vi "Start Sync.vi"(8 "error in":errorcluster, 10 "measurement plugin service in":refnum<class "Measurement Plugin Service.lvclass">, 11 "measurement service v1 in":refnum<class "Measurement Service V1.lvclass">) -> (0 "error out":errorcluster, 3 "measurement service v1 out":refnum<class "Measurement Service V1.lvclass">)   [LabVIEW 2020, in "Measurement Plugin Measurement Server.lvlib" / "Measurement Service V1.lvclass"]
uses:
  Measurement Service V1.lvclass
  C:/dev/measurementlink-labview/Source/Runtime/Measurement Plugin Measurement Server/IMeasurement Service/IMeasurement Service.lvclass
  Measurement Plugin Service/Measurement Plugin Service.lvclass
  Measurement Service V1.lvclass/Measurement Service V1.ctl
  Measurement Plugin Measurement Server Internal/RPC Service/MeasurementService/MeasurementServiceBaseV1.lvclass
  IMeasurement Service/IMeasurement Service.lvclass
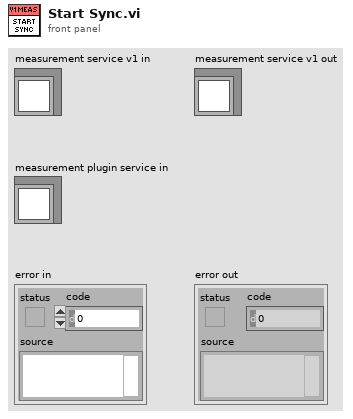
[diagram p1: front panel]
types:
  T1 = typedef "grpc-lvsupport-release.lvlib/grpcId.ctl" = u64
  T2 = typedef "Measurement Plugin Measurement Server.lvlib/Get Metadata Response.ctl" = cluster{"measurement details":T3, "measurement signature":T4, "user interface details":T9[]}
  T3 = typedef "Measurement Plugin Measurement Server.lvlib/Measurement Details.ctl" = cluster{"display name":string, "version":string}
  T4 = typedef "Measurement Plugin Measurement Server.lvlib/Measurement Signature.ctl" = cluster{"configuration parameters message type":string, "configuration parameters":T5[], "configuration defaults":T7, "outputs message type":string, "outputs":T8[]}
  T5 = typedef "Measurement Plugin Measurement Server.lvlib/Configuration Parameter.ctl" = cluster{"field number":i32, "type":i32, "name":string, "repeated":bool, "annotations":T6[], "message type":string}
  T6 = typedef "Measurement Plugin Measurement Server.lvlib/Parameter Annotations Entry.ctl" = cluster{"key":string, "value":string}
  T7 = typedef "grpc-lvsupport-release.lvlib/Any.ctl" = cluster{"Type Url":string, "Bytes":u8[]}
  T8 = typedef "Measurement Plugin Measurement Server.lvlib/Output Parameter.ctl" = cluster{"field number":i32, "type":i32, "name":string, "repeated":bool, "annotations":T6[], "message type":string}
  T9 = typedef "Measurement Plugin Measurement Server.lvlib/User Interface Details.ctl" = cluster{"file url":string}
  T10 = typedef "Measurement Plugin Measurement Server Internal.lvlib/ni_measurementlink_measurement_v1_GetMetadataResponse.ctl" = cluster{"measurement_details":T11, "measurement_signature":T12, "user_interface_details":T18[]}
  T11 = typedef "Measurement Plugin Measurement Server Internal.lvlib/ni_measurementlink_measurement_v1_MeasurementDetails.ctl" = cluster{"display_name":string, "version":string}
  T12 = typedef "Measurement Plugin Measurement Server Internal.lvlib/ni_measurementlink_measurement_v1_MeasurementSignature.ctl" = cluster{"configuration_parameters_message_type":string, "configuration_parameters":T13[], "configuration_defaults":T16, "outputs_message_type":string, "outputs":T17[]}
  T13 = typedef "Measurement Plugin Measurement Server Internal.lvlib/ni_measurementlink_measurement_v1_ConfigurationParameter.ctl" = cluster{"field_number":i32, "type":T14, "name":string, "repeated":bool, "annotations":T15[]}
  T14 = typedef "Measurement Plugin Measurement Server Internal.lvlib/google_protobuf_Field_Kind.ctl" = enum32{"TYPE_UNKNOWN", "TYPE_DOUBLE", "TYPE_FLOAT", "TYPE_INT64", "TYPE_UINT64", "TYPE_INT32", "TYPE_FIXED64", "TYPE_FIXED32", "TYPE_BOOL", "TYPE_STRING", "TYPE_GROUP", "TYPE_MESSAGE", "TYPE_BYTES", "TYPE_UINT32", "TYPE_ENUM", "TYPE_SFIXED32", "TYPE_SFIXED64", "TYPE_SINT32", "TYPE_SINT64"}
  T15 = typedef "Measurement Plugin Measurement Server Internal.lvlib/ni_measurementlink_measurement_v1_ConfigurationParameter_AnnotationsEntry.ctl" = cluster{"key":string, "value":string}
  T16 = typedef "Measurement Plugin Measurement Server Internal.lvlib/google_protobuf_Any.ctl" = cluster{"type_url":string, "value":u8[]}
  T17 = typedef "Measurement Plugin Measurement Server Internal.lvlib/ni_measurementlink_measurement_v1_Output.ctl" = cluster{"field_number":i32, "type":T14, "name":string, "repeated":bool}
  T18 = typedef "Measurement Plugin Measurement Server Internal.lvlib/ni_measurementlink_measurement_v1_UserInterfaceDetails.ctl" = cluster{"file_url":string}
  T19 = typedef "Measurement Plugin Measurement Server Internal.lvlib/ni_measurementlink_measurement_v1_MeasureRequest.ctl" = cluster{"configuration_parameters":T16, "pin_map_context":T20}
  T20 = typedef "Measurement Plugin Measurement Server Internal.lvlib/ni_measurementlink_PinMapContext.ctl" = cluster{"pin_map_id":string, "sites":i32[]}
  T21 = typedef "Measurement Plugin Measurement Server.lvlib/Measure Response.ctl" = cluster{"outputs":T16}
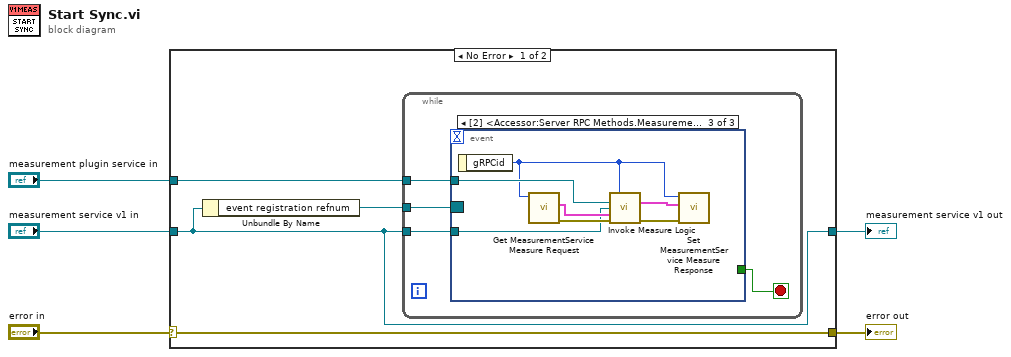
[diagram p0: block diagram]
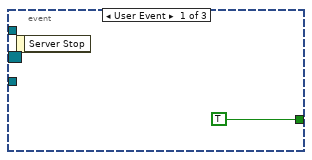
[diagram p2: hidden frame]
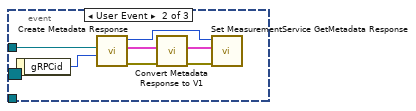
[diagram p3: hidden frame]
diagram:
  n1 = case shown="No Error" "error in" {
    selector: "error in" -> [w6 w30]
    tunnel: [w6 w30] -> w3
    tunnel: "measurement plugin service in" -> [w9 _]
    tunnel: "measurement service v1 in" -> [w8 w29]
    tunnel: [w8 w29] -> w1
    frame No Error {
      n2 = Unbundle By Name(w8) -> ("event registration refnum"=w7:refnum<event-registration>)
      n3 = while {
        tunnel: w7 -> [w13]
        tunnel: w9 -> [w12]
        tunnel: w8 -> [w10]
        stop <- w11 stop-if-true
        n4 = event "RPC Methods Event Structure" shown="[2] <Accessor:Server RPC Methods.MeasurementService Measure gRPC UE>: User Event" {
          selector: w13 -> [_ _ _]
          dyn-events: _ -> [_ _ _]
          timeout: _ -> [_ _ _]
          tunnel: [TRUE _ _] -> w11
          tunnel: w12 -> [_ w19 w27]
          tunnel: w10 -> [_ _ w22]
          event User Event {
            n5 = event-data() -> ()  [unwired: 1 in, 1 out]
          }
          event User Event {
            n6 = event-data() -> ("gRPCid"=w20:T1)  [unwired: 1 in]
            n7 = call "Create Metadata Response.vi"("gRPC ID"=w20, "measurement plugin service in"=w19) -> ("error out"=w18:errorcluster, "get metadata response"=w16:T2, "gRPC ID out"=w21:T1)  [unwired: 7 in]
            n8 = call "Convert Metadata Response to V1.vi"("error in"=w18, "get metadata response generic in"=w16) -> ("error out"=w17:errorcluster, "get metadata response v1 out"=w15:T10)  [unwired: 8 in]
            n9 = call "Set MeasurementService GetMetadata Response.vi"("error in (no error)"=w17, "Message Data"=w15, "gRPCid in"=w21) -> ()  [unwired: 8 in, 1 out]
          }
          event User Event {
            n10 = event-data() -> ("gRPCid"=w23:T1)  [unwired: 1 in]
            n11 = call "Get MeasurementService Measure Request.vi"("gRPCid"=w23) -> ("error out"=w25:errorcluster, "Message Data"=w24:T19)  [unwired: 8 in, 1 out]
            n12 = call "Invoke Measure Logic.vi"("gRPC ID in"=w23, "measurement plugin service in"=w27, "measurement service in"=w22, "measure request"=w24, "error in"=w25) -> ("measure response"=w26:T21, "error out"=w28:errorcluster)  [unwired: 9 in]
            n13 = call "Set MeasurementService Measure Response.vi"("error in (no error)"=w28, "Message Data"=w26, "gRPCid in"=w23) -> ()  [unwired: 8 in, 1 out]
          }
        }
      }
    }
    frame Error {
    }
  }
  "error out" <- w3
  "measurement service v1 out" <- w1
